vi "WildDrive_v2.vi"(9 "Super_Turn":bool, 10 "Turn":dbl, 11 "Speed":dbl) -> (2 "Right Side Power":dbl, 3 "Left Side Power":dbl)   [LabVIEW 2018]
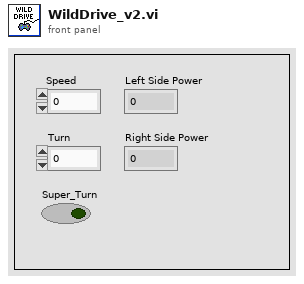
[diagram p1: front panel]
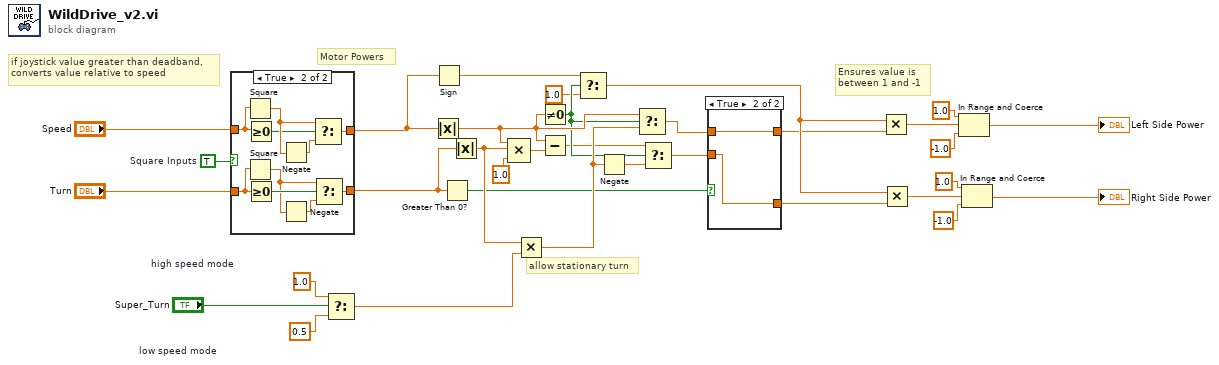
[diagram p0: block diagram]
diagram:
  w32 = 0.5  # low speed mode
  w31 = 1.0  # high speed mode
  w7 = TRUE  # Square Inputs
  # "Ensures value is \nbetween 1 and -1"
  # "if joystick value greater than deadband,\nconverts value relative to speed"
  # "allow stationary turn"
  # "Motor Powers"
  n1 = case shown="True" w7 {
    tunnel: [w34 w45] -> w2
    tunnel: [w35 w44] -> w1
    tunnel: "Turn" -> [w34 w43]
    tunnel: "Speed" -> [w35 w42]
    frame False {
    }
    frame True {
      n2 = Square(x=w42) -> (x^2=w37:dbl)
      n3 = Square(x=w43) -> (x^2=w40:dbl)
      n4 = Greater Or Equal To 0?(x=w42) -> (x >= 0?=w36:bool)
      n5 = Greater Or Equal To 0?(x=w43) -> (x >= 0?=w41:bool)
      n6 = Negate(x=w37) -> (-x=w38:dbl)
      n7 = Negate(x=w40) -> (-x=w39:dbl)
      n8 = Select(t=w37, s=w36, f=w38) -> (s? t:f=w44:dbl)
      n9 = Select(t=w40, s=w41, f=w39) -> (s? t:f=w45:dbl)
    }
  }
  n10 = Select(t=w31, s="Super_Turn", f=w32) -> (s? t:f=w33:dbl)
  n11 = Absolute Value(x=w1) -> (abs(x)=w16:dbl)
  n12 = Sign(1:w1) -> (0:w9:dbl)
  n13 = Greater Than 0?(x=w2) -> (x > 0?=w3:bool)
  n14 = Absolute Value(x=w2) -> (abs(x)=w8:dbl)
  n15 = Compound Arithmetic op=MULTIPLY(w16, w8, 1.0 ("y")) -> (w11:dbl)
  n16 = Multiply(x=w8, y=w33) -> (x*y=w17:dbl)
  n17 = Not Equal To 0?(x=w16) -> (x != 0?=w15:bool)
  n18 = Subtract(x=w16, y=w11) -> (x-y=w13:dbl)
  n19 = Select(t=w9, s=w15, f=1.0) -> (s? t:f=w26:dbl)
  n20 = Negate(x=w17) -> (-x=w18:dbl)
  n21 = Select(t=w16, s=w15, f=w17) -> (s? t:f=w14:dbl)
  n22 = Select(t=w13, s=w15, f=w18) -> (s? t:f=w12:dbl)
  n23 = case shown="True" w3 {
    tunnel: w12 -> [w46 w49]
    tunnel: [w46 w48] -> w25
    tunnel: w14 -> [w47 w48]
    tunnel: [w47 w49] -> w27
    frame False {
    }
    frame True {
    }
  }
  n24 = Multiply(x=w26, y=w25) -> (x*y=w19:dbl)
  n25 = Multiply(x=w26, y=w27) -> (x*y=w24:dbl)
  n26 = In Range and Coerce(upper limit=1.0, x=w19, lower limit=-1.0) -> (coerced(x)=→"Left Side Power":dbl)  [unwired: 1 out]
  n27 = In Range and Coerce(upper limit=1.0, x=w24, lower limit=-1.0) -> (coerced(x)=→"Right Side Power":dbl)  [unwired: 1 out]
